vi "IV getadc.vi"(8 "error in (no error)":errorcluster, 10 "value":dbl, 11 "channr":i32) -> (0 "error out":errorcluster, 1 "return type":i32, 2 "value out":dbl, 3 "channr out":i32)   [LabVIEW 2020, in "IVIUM_remdriver.lvlib"]
uses:
  IVIUM_remdriver.lvlib
  SEC Software V4.9/Dependencies/Drivers and Aux files/IVIUM/IVIUM_remdriver.dll
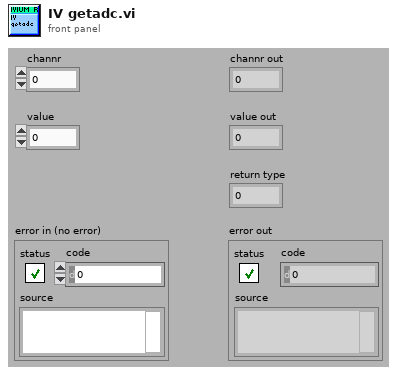
[diagram p1: front panel]
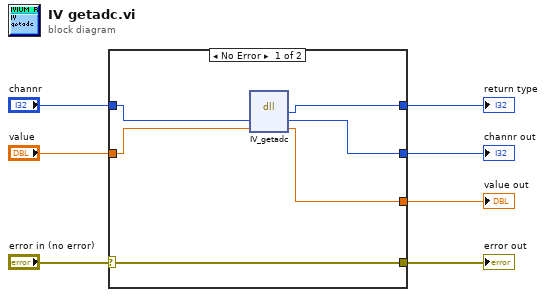
[diagram p0: block diagram]
diagram:
  n1 = case shown="No Error" "error in (no error)" {
    selector: "error in (no error)" -> [w13 w16]
    tunnel: [w13 w16] -> w6
    tunnel: [w12 _] -> w5
    tunnel: "channr" -> [w11 w15]
    tunnel: [w10 w15] -> w3
    tunnel: "value" -> [w9 w14]
    tunnel: [w8 w14] -> w1
    frame No Error {
      n2 = dll-call lib="C:/Users/Benj/Desktop/SEC Software V4.9/Dependencies/Drivers and Aux files/IVIUM/IVIUM_remdriver.*" fn="IV_getadc"("channr"=w11, "value"=w9) -> (w12:i32, "channr"=w10:i32, "value"=w8:dbl)  [unwired: 3 in, 2 out]
    }
    frame Error {
    }
  }
  "return type" <- w5
  "channr out" <- w3
  "value out" <- w1
  "error out" <- w6
